vi "Configure Specific Limit Test.vi"(0 "VISA resource name":refnum<visa-resource-name>, 1 "Enable Limit Test  (T:Enable)":bool=TRUE, 5 "Limit Test Number (2)":u16=2 min=1 max=2 step=1, 7 "Lower Limit (0)":dbl, 9 "Upper Limit (1)":dbl=1.0, 11 "error in (no error)":errorcluster, 12 "Function (0: Volts)":u16(ring) items=["Volts", "Current", "Resistance"]) -> (4 "VISA resource name out":refnum<visa-resource-name>, 15 "error out":errorcluster)   [LabVIEW 2022 SP3, in "Keithley 2450.lvlib"]
doc: "Configures limit testing settings, such as the enabling or disabling limit test, setting upper and lower limit."
uses:
  Keithley 2450.lvlib
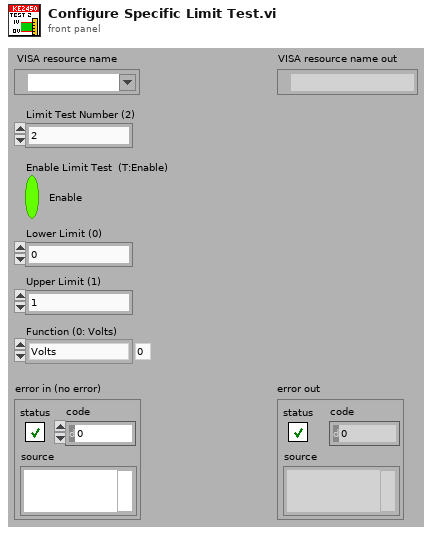
[diagram p1: front panel]
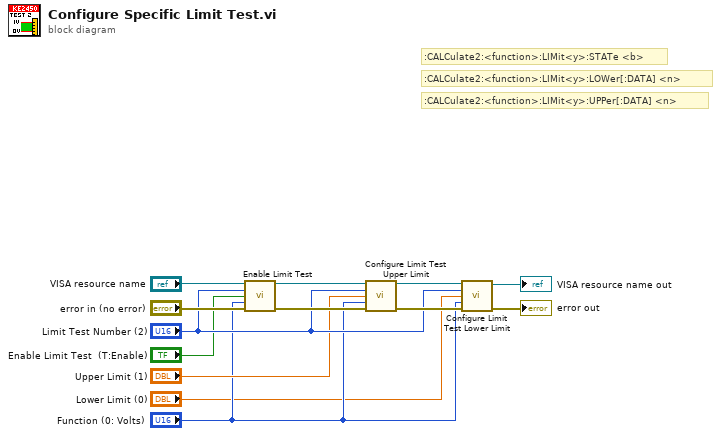
[diagram p0: block diagram]
diagram:
  # ":CALCulate2:<function>:LIMit<y>:UPPer[:DATA] <n>"
  # ":CALCulate2:<function>:LIMit<y>:LOWer[:DATA] <n>"
  # ":CALCulate2:<function>:LIMit<y>:STATe <b>"
  n1 = call "Enable Limit Test.vi"("VISA resource name"="VISA resource name", "Limit Test Number (2)"="Limit Test Number (2)", "Enable Limit Test  (T:Enable)"="Enable Limit Test  (T:Enable)", "Function (0: Volts)"="Function (0: Volts)", "error in (no error)"="error in (no error)") -> ("VISA resource name out"=w8:refnum<visa-resource-name>, "error out"=w12:errorcluster)  [unwired: 9 in]
  n2 = call "Configure Limit Test Upper Limit.vi"("VISA resource name"=w8, "Limit Test Number (1)"="Limit Test Number (2)", "Upper Limit (1)"="Upper Limit (1)", "Function (0: Volts)"="Function (0: Volts)", "error in (no error)"=w12) -> ("VISA resource name out"=w7:refnum<visa-resource-name>, "error out"=w11:errorcluster)  [unwired: 9 in]
  n3 = call "Configure Limit Test Lower Limit.vi"("VISA resource name"=w7, "Limit Test Number (1)"="Limit Test Number (2)", "Lower Limit (-1.0)"="Lower Limit (0)", "Function (0: Volts)"="Function (0: Volts)", "error in (no error)"=w11) -> ("VISA resource name out"=→"VISA resource name out":refnum<visa-resource-name>, "error out"=→"error out":errorcluster)  [unwired: 9 in]
